vi "TC test USB4718 v1.vi"() -> ()   [LabVIEW 2013]
uses:
  <vilib>/Platform/TimedLoop/XDataNode/timing_clust.ctl
  <vilib>/Platform/TimedLoop/XDataNode/nitl_modes.ctl
  <vilib>/Platform/TimedLoop/XDataNode/wakeup.ctl
  <vilib>/platform/TimedLoop/XDataNode/XDataNode.xnode
  <vilib>/Platform/TimedLoop/XDataNode/XDNodeRunTimeDep.lvlib
panel:
  out "T3":dbl
  out "T7":dbl
  out "cycle":bool
  out "Waveform Chart":dynamicdata(graph)
  out "T2":dbl
  out "T1":dbl
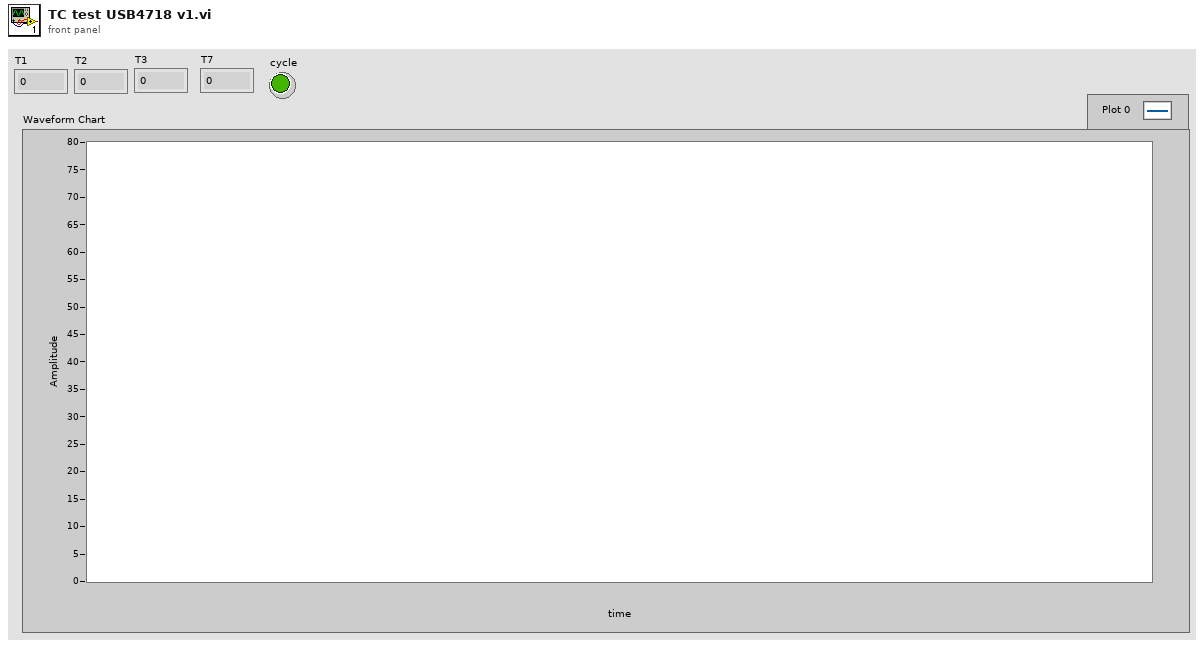
[diagram p1: front panel]
types:
  T1 = typedef "XDNodeRunTimeDep.lvlib/timing_clust.ctl" = cluster{"Expected End [f-1]":u64, "Actual End [f-1]":u64, "Finished Late? [f-1]":bool, "Expected End [i-1]":u64, "Actual End [i-1]":u64, "Finished Late? [i-1]":bool, "Expected Start [i]":u64, "Actual Start [i]":u64, "Expected Start [f]":u64, "Actual Start [f]":u64, "Source Name":string, "Structure Name":string, "Period":i64, "Deadline":i64, "Offset":i64, "Start":i64, "Priority":i32, "Timeout":i32, "Mode":T2, "Wakeup Reason":T3, "Error":errorcluster, "Source Type":string, "Secondary Source Type":string, "Global End Time":u64, "Global Start Time":u64, "Frame Duration":u64, "Iteration Duration":u64, "Assigned CPU":i32, "I/O Scan Engine Mode":u32}
  T2 = typedef "XDNodeRunTimeDep.lvlib/nitl_modes.ctl" = enum32{"No Change", "Process missed periods, maintain original phase", "Discard missed periods, maintain original phase", "Process missed periods, ignore original phase", "Discard missed periods, ignore original phase"}
  T3 = typedef "XDNodeRunTimeDep.lvlib/wakeup.ctl" = enum32{"Normal", "Aborted", "Asynchronous wakeup", "Timing source error", "Timed loop error", "Timeout"}
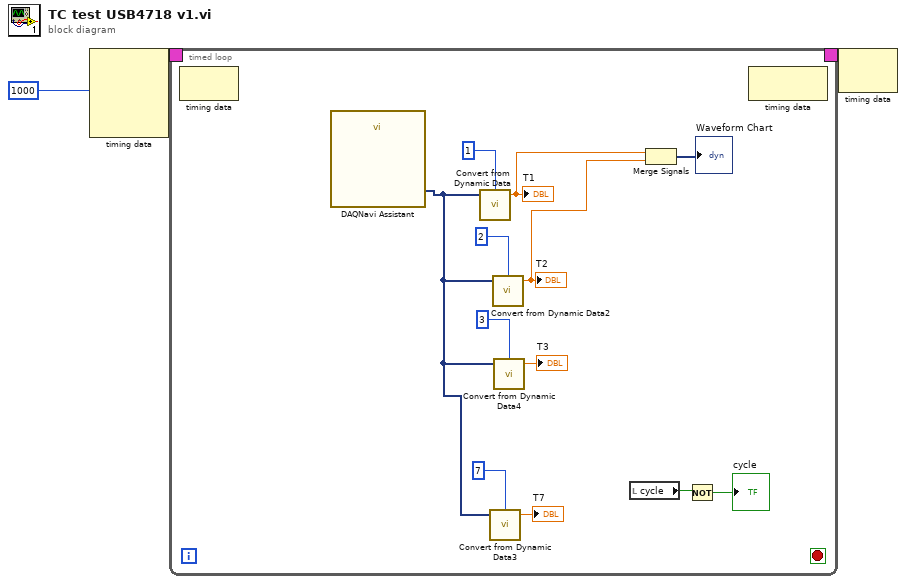
[diagram p0: block diagram]
diagram:
  n1 = node-c288(1000) -> (w3:T1)  [unwired: 3 in]
  n2 = timed-loop {
    timing: w3 -> [_]
    timing-out: [_] -> w2
    stop <- _ stop-if-true
    n3 = node-c288() -> ()  [unwired: 1 in, 1 out]
    n4 = call "DAQNavi Assistant"() -> ("data out(DDT)"=w6:dynamicdata)  [unwired: 26 in, 1 out]
    n5 = call "Convert from Dynamic Data"("Dynamic Data Type"=w6, "Channel"=1) -> ("Scalar"=w13:dbl)  [unwired: 2 in]
    "T1" <- w13
    n6 = call "Convert from Dynamic Data3"("Dynamic Data Type"=w6, "Channel"=7) -> ("Scalar"=→"T7":dbl)  [unwired: 2 in]
    n7 = call "Convert from Dynamic Data2"("Dynamic Data Type"=w6, "Channel"=2) -> ("Scalar"=w12:dbl)  [unwired: 2 in]
    "T2" <- w12
    n8 = call "Convert from Dynamic Data4"("Dynamic Data Type"=w6, "Channel"=3) -> ("Scalar"=→"T3":dbl)  [unwired: 2 in]
    n9 = local read "cycle"() -> (w9:bool)
    n10 = Merge Signals(w13, w12) -> (→"Waveform Chart":dynamicdata)
    n11 = Not(x=w9) -> (.not. x?=→"cycle":bool)
    n12 = node-c288() -> ()  [unwired: 1 in, 1 out]
  }
  n13 = node-c288(w2) -> ()  [unwired: 1 out]
